vi "Completed Test Case.vi"(10 "Test Case Result":T1, 11 "Test Suite In":refnum<class "LUnit Test Suite.lvclass">) -> (3 "Test Suite Out":refnum<class "LUnit Test Suite.lvclass">)   [LabVIEW 2020, in "LUnit Test Suite.lvclass"]
doc: "Generate test case rusults and increment current test."
uses:
  LUnit Test Suite.lvclass
  Result Types/Case Result/Test Case Result.ctl
  Result Types/Method Result/Method Result.ctl
  Rewrite Project/Result/Status.ctl
  Result Types/Assertion Result/Assertion Result.ctl
  Result Types/Assertion Result/Public/TypeDefs/Assertion Type.ctl
  LUnit Test Suite.lvclass/LUnit Test Suite.ctl
  Result Types/Case Result/Public/Read Status.vi
  Result Types/Suite Results/Private/Merge Status.vi
  Result Types/Case Result/Private/Merge Status.vi
  Result Types/Method Result/Public/Read Status.vi
  Result Types/Suite Results/Test Suite Result.lvlib
  Result Types/Assertion Result/Assertion Result.lvlib
  Result Types/Method Result/Method Result.lvlib
  Result Types/Case Result/Test Case Result.lvlib
  Rewrite Project/Result/Result.lvlib
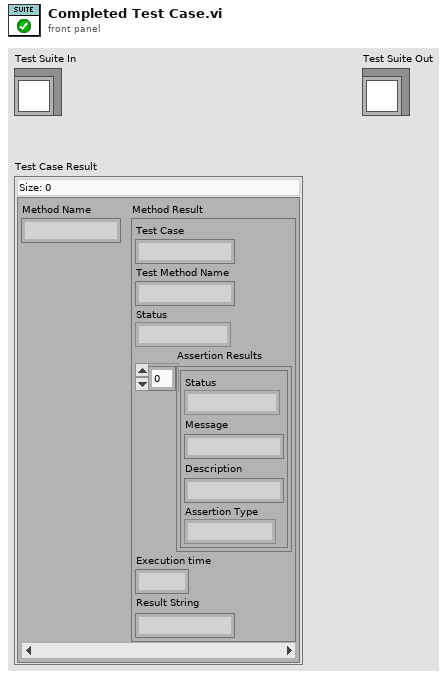
[diagram p1: front panel]
types:
  T1 = typedef "Test Case Result.lvlib/Test Case Result.ctl" = map{string, T2}
  T2 = typedef "Method Result.lvlib/Method Result.ctl" = cluster{"Test Case":string, "Test Method Name":string, "Status":T3, "Assertion Results":T4[], "Execution time":dbl, "Result String":string}
  T3 = typedef "Result.lvlib/Status.ctl" = enum16{"Pass", "Fail", "Error", "Skipped", "Setup Error", "Broken", "Teardown Error"}
  T4 = typedef "Assertion Result.lvlib/Assertion Result.ctl" = cluster{"Status":T3, "Message":string, "Description":string, "Assertion Type":T5}
  T5 = typedef "Result.lvlib/Assertion Type.ctl" = enum16{"None", "Pass", "Fail", "Skip", "Pass if Equal", "Fail if Equal", "Pass if Error", "Fail if Error", "Pass if", "Fail if"}
  T6 = typedef "Test Suite Result.lvlib/Test Suite Result.ctl" = cluster{"Test Suite ID":string, "Name":string, "Hostname":string, "Status":T7, "Execution time":dbl, "Start Time":timestamp, "Case Results":T1[]}
  T7 = typedef "Assertion Result.lvlib/Status.ctl" = enum16{"Pass", "Fail", "Error", "Skipped", "Setup Error", "Broken", "Teardown Error"}
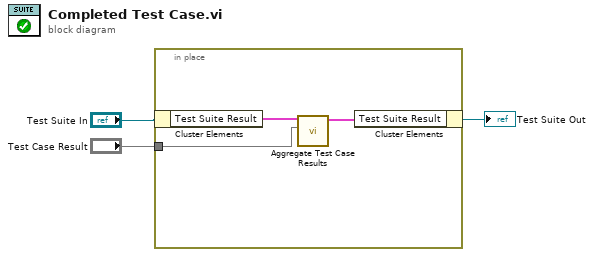
[diagram p0: block diagram]
diagram:
  n1 = in-place {
    in-place-border: "Test Case Result" -> [w4]
    n2 = in-place-cluster #1("Test Suite In") -> ("Test Suite Result"=w6:T6)
    n3 = call "Aggregate Test Case Results.vi"("Test Case Result"=w4, "Test Suite Result In"=w6) -> ("Test Suite Result Out"=w5:T6)  [unwired: 9 in]
    n4 = in-place-cluster #1("Test Suite Result"=w5) -> (→"Test Suite Out":refnum<class "LUnit Test Suite.lvclass">)
  }
